vi "Apply Transformations.vi"(8 "error in (no error)":errorcluster, 11 "Tool Object in":refnum<class "Tool Object.lvclass">) -> (0 "error out":errorcluster, 3 "Tool Object out":refnum<class "Tool Object.lvclass">)   [LabVIEW 2019, in "Tool Object.lvclass"]
uses:
  Tool Object.lvclass
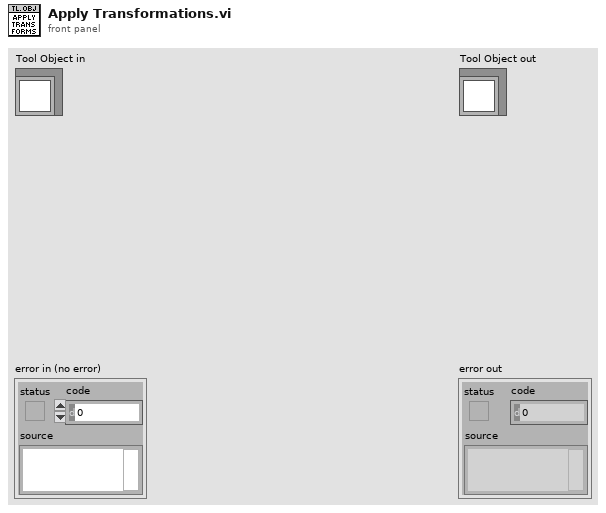
[diagram p1: front panel]
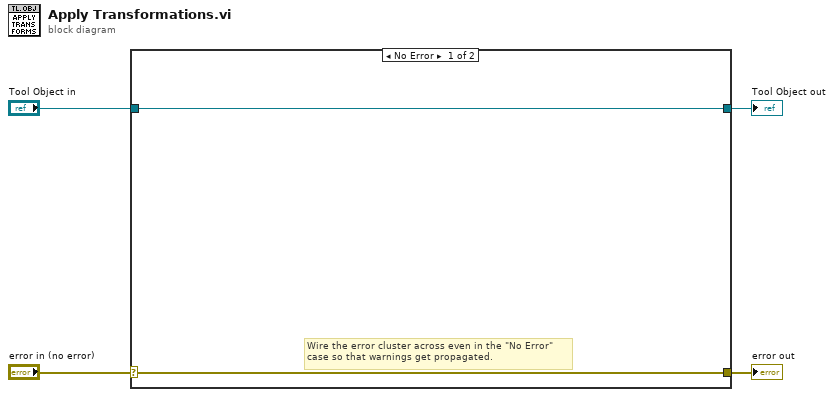
[diagram p0: block diagram]
diagram:
  n1 = case shown="No Error" "error in (no error)" {
    selector: "error in (no error)" -> [w5 w8]
    tunnel: [w5 w8] -> w3
    tunnel: [w6 w7] -> w1
    tunnel: "Tool Object in" -> [w6 w7]
    frame No Error {
      # "Wire the error cluster across even in the \"No Error\"\ncase so that warnings get propagated."
    }
    frame Error {
    }
  }
  "error out" <- w3
  "Tool Object out" <- w1
